vi "CPP_SpectraFit.vi"() -> (5 "Plug in titles":string[](array[string]), 7 "Plug in values":string[](array[string]))   [LabVIEW 2010]
uses:
  Controls/Instrument_Array.ctl
  Controls/Post_Process.ctl
  Controls/Graph_Type.ctl
  Globals/Meas_global.vi
  Globals/Plug_in_data_global.vi
panel:
  out "dF/ Hz":dbl
  in  "Show Smooth":bool=TRUE
  in  "Save Spectra?":bool
  in  "Desired number of samples per block":i32=32767
  in  "Calculate Spectra and Histogram?":bool=TRUE
  out "Spectra":cluster{dbl, dbl, "Spectrum output array":dbl[]}(graph)
  in  "Averaging samples":i32=1 min=1 max=1000
  in  "Spectra Index (from ALL channels)":i32
  out "Waveform Graph":dbl[][](graph)
  in  "Channels to Plot":i32[](array[ring])=[0] items=["Pitot (Uref)", "HW (Uhw)", "Gen (Trav)", "Save Nothing"]
  # "Run this VI to update the channel names"
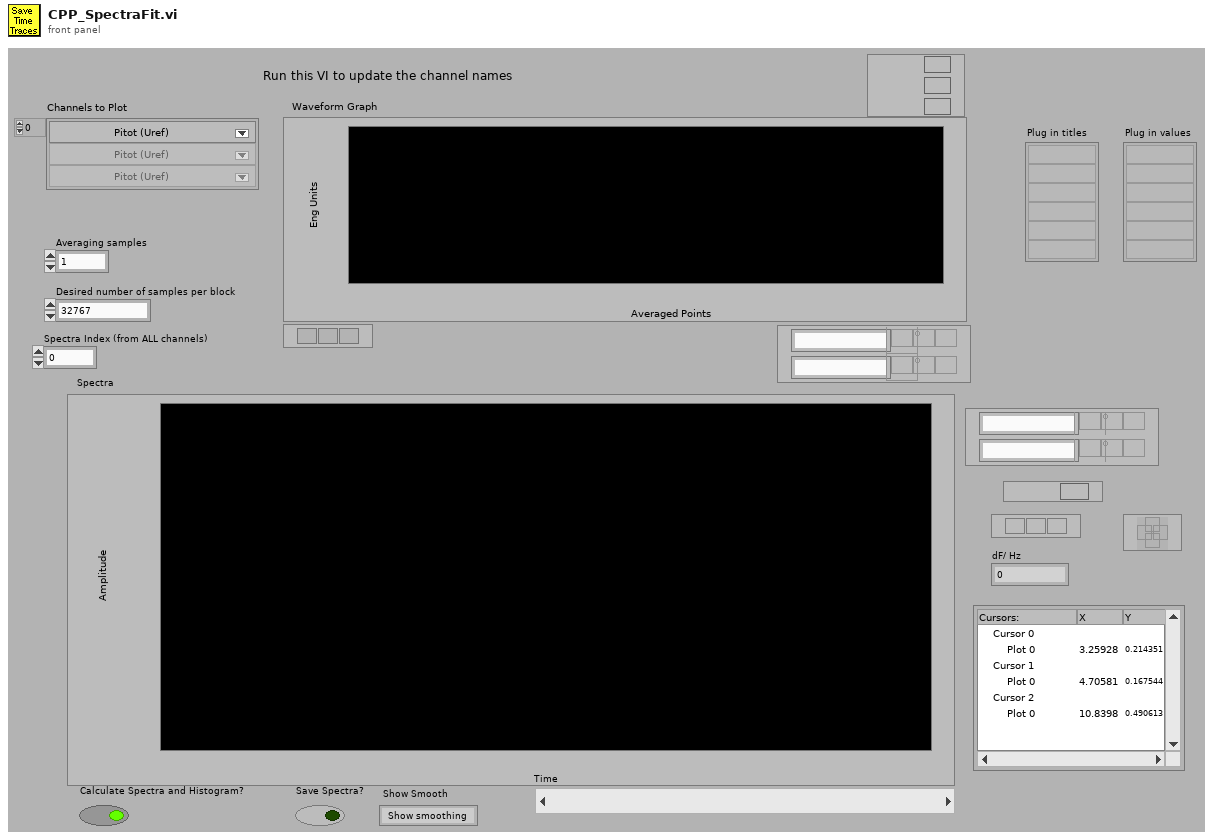
[diagram p1: front panel]
types:
  T1 = typedef "Analysis_info_cluster.ctl" = cluster{"Colour":u32, "Inst type":T2, "Inst name":string, "Symbol":string, "Code name":string, "Extra Info":string, "Inst Array":T3, "Index":i32, "Voltage Index":i32, "Extra Titles":string[], "Extra Values":string[]}
  T2 = typedef "Inst_type.ctl" = enum16{"Propeller anemometer", "Raw voltage", "Pressure Transducer", "Pitot-static tube", "Preston tube", "Hot wire", "Cross wire 1", "Cross wire 2", "Generic Linear", "Generic Polynomial", "Generic BackPoly", "Fast FID", "Thermocouple", "Cold wire", "Pulsed Wire", "LDA Vel", "LDA Tran time", "LDA Arr time"}
  T3 = typedef "Instrument_Array.ctl" = enum16{"PWA", "LDA", "Analogue"}
  T4 = typedef "Post_Process.ctl" = enum16{"Take New Data", "Post Process Raw Data File"}
  T5 = typedef "Graph_Type.ctl" = enum16{"Show no graph", "Voltage trace", "Velocity trace", "Vel histogram", "Spectrum", "f.E(f) v Log f", "Auto-Corr"}
  T6 = cluster{"Plot 1":u16, "Plot 2":u16, "Save graph":u16, "Plot Type":T5}
  T7 = cluster{dbl, dbl, "Spectrum output array":dbl[]}[]
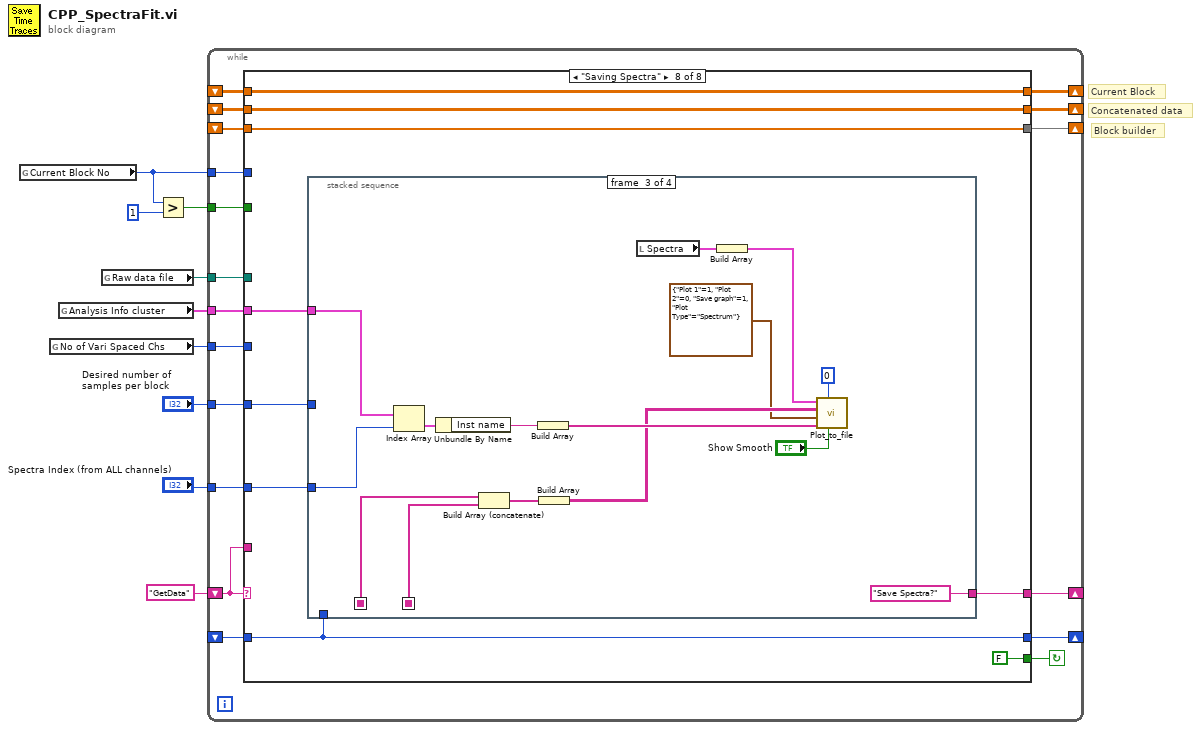
[diagram p0: block diagram]
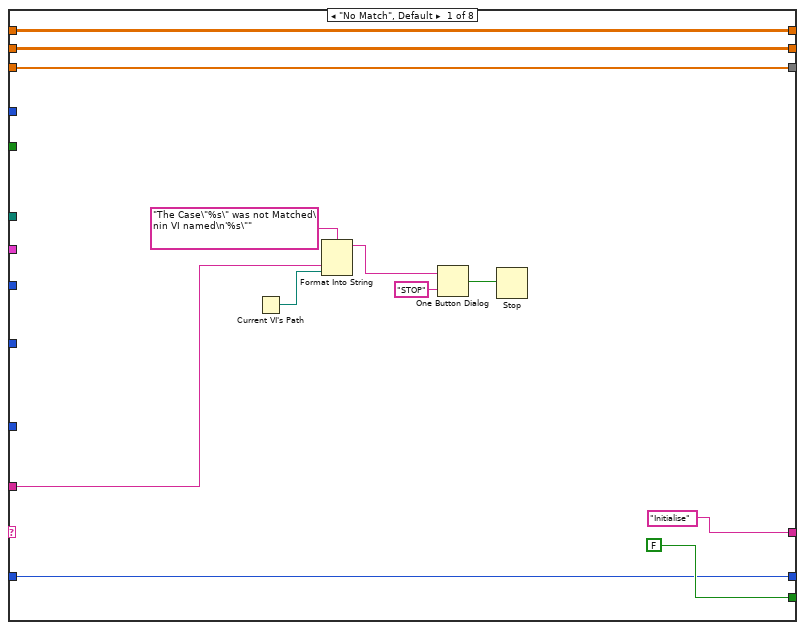
[diagram p2: hidden frame]
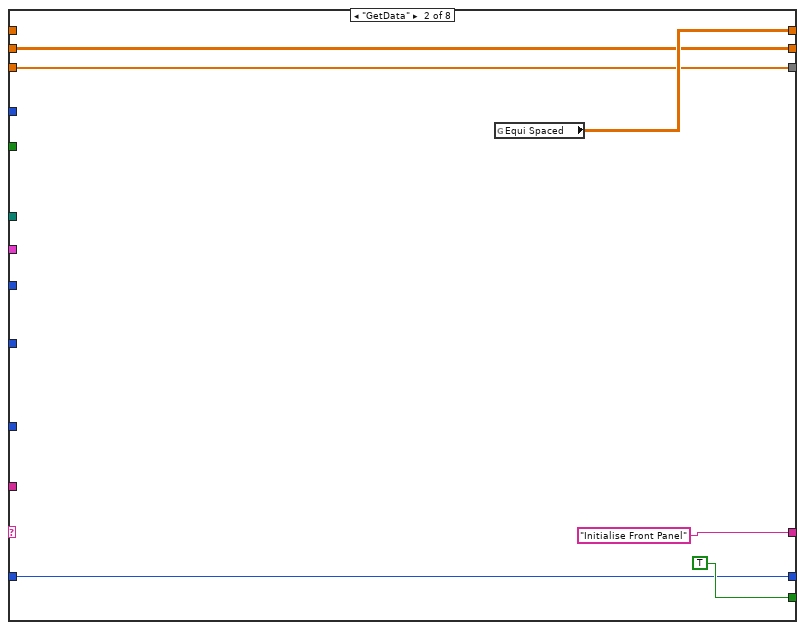
[diagram p3: hidden frame]
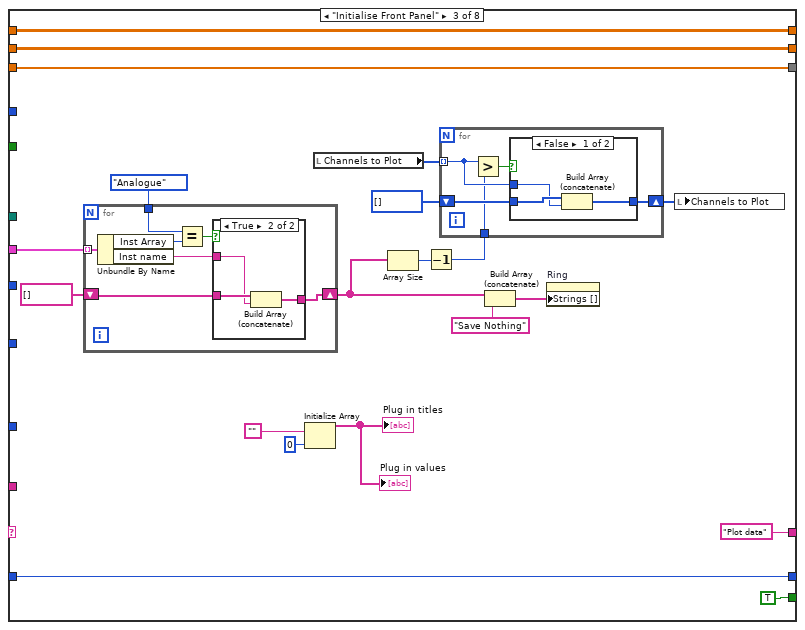
[diagram p4: hidden frame]
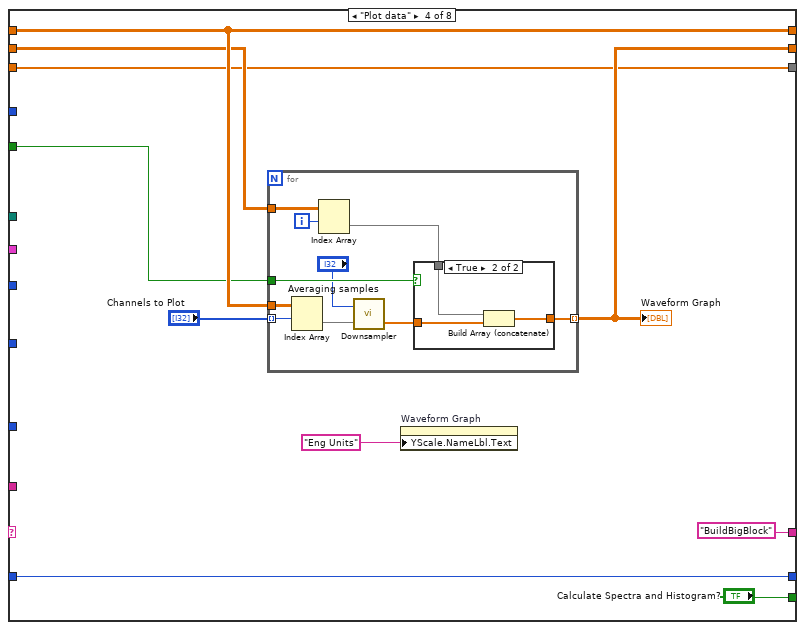
[diagram p7: hidden frame]
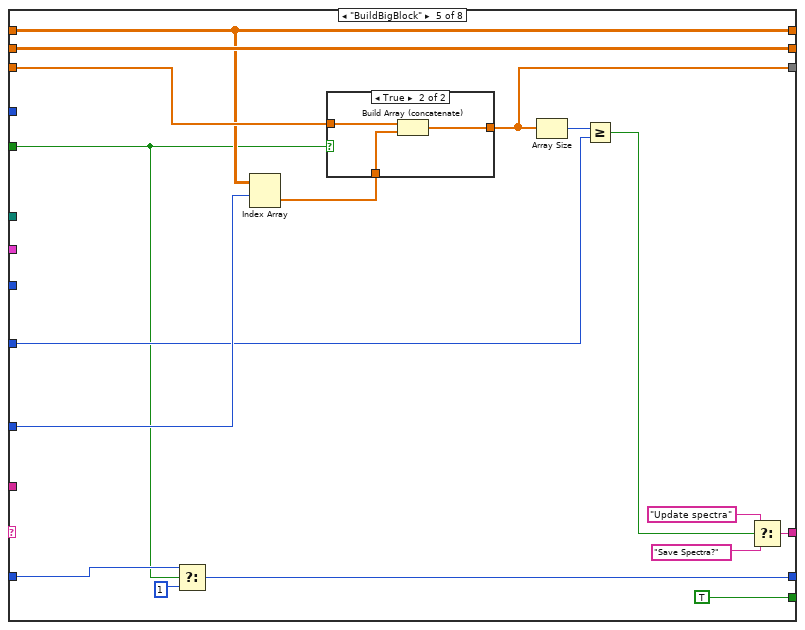
[diagram p9: hidden frame]
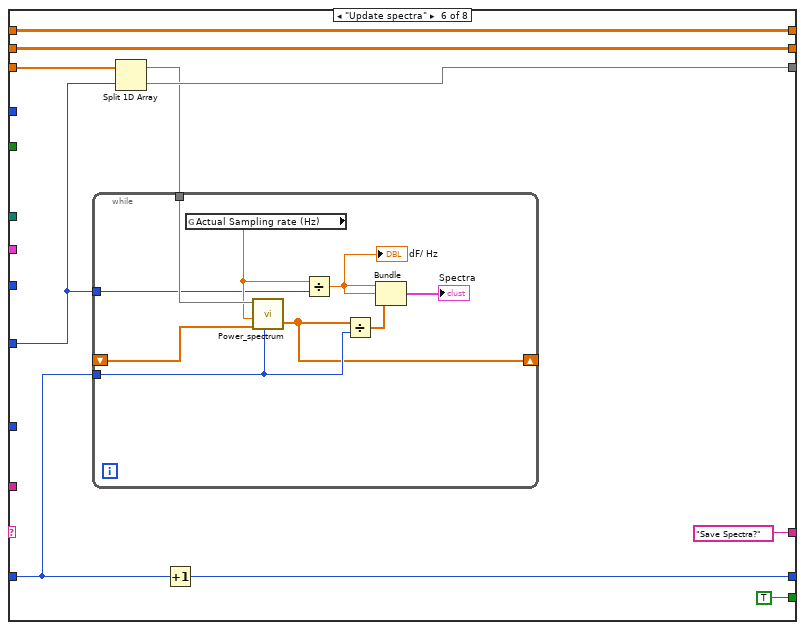
[diagram p11: hidden frame]
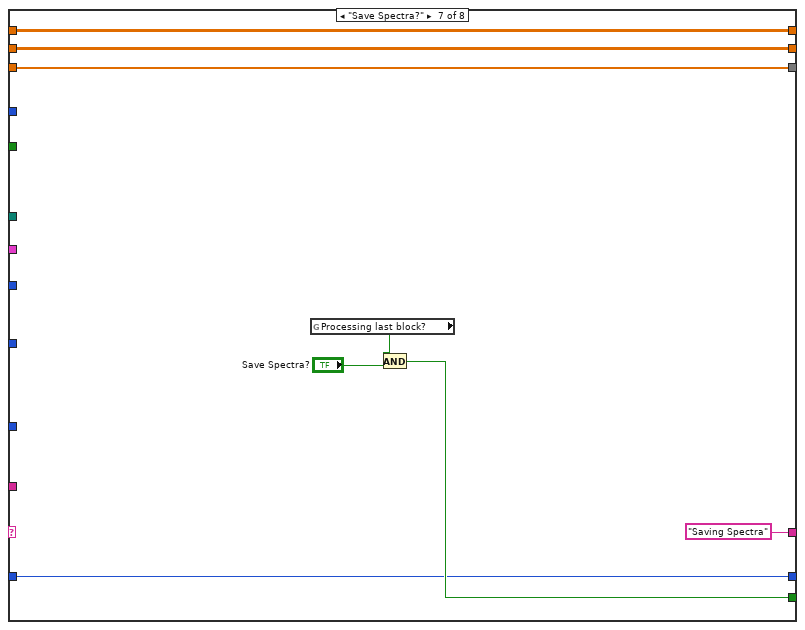
[diagram p12: hidden frame]
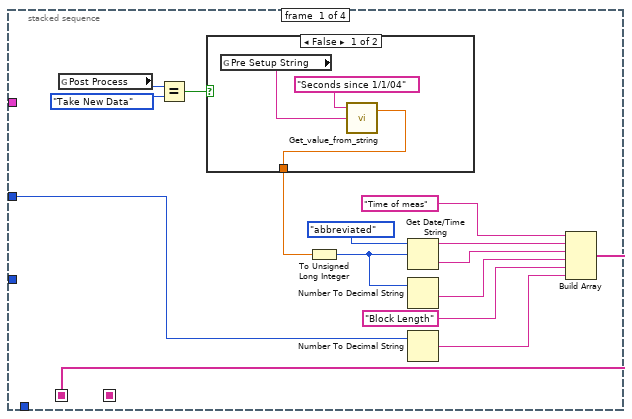
[diagram p13: hidden frame]
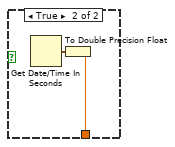
[diagram p14: hidden frame]
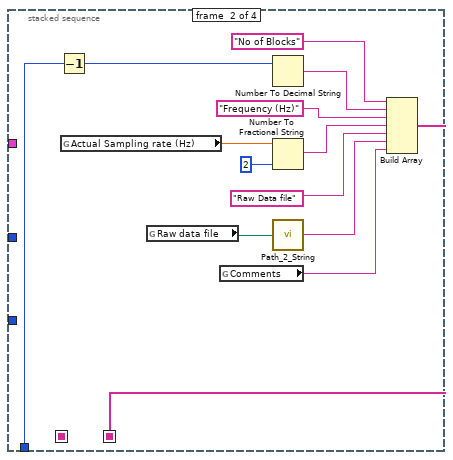
[diagram p15: hidden frame]
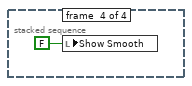
[diagram p16: hidden frame]
diagram:
  # "Block builder"
  # "Concatenated data"
  # "Current Block"
  n1 = global read "Meas_global.vi" "Current Block No"() -> (w6:i32)
  n2 = global read "Meas_global.vi" "No of Vari Spaced Chs"() -> (w4:i32)
  n3 = global read "Meas_global.vi" "Analysis Info cluster"() -> (w5:T1[])
  n4 = global read "Meas_global.vi" "Raw data file"() -> (w8:path)
  n5 = Greater?(x=w6, y=1) -> (0:w3:bool)
  n6 = while {
    shift-left: "GetData" -> [w25]
    shift-right: [w26] -> _
    tunnel: w8 -> [w24]
    tunnel: w3 -> [w23]
    tunnel: w6 -> [w22]
    tunnel: w5 -> [w21]
    tunnel: w4 -> [w20]
    shift-right: [w19] -> _
    shift-left: _ -> [w18]
    shift-right: [w16] -> _
    shift-left: _ -> [w17]
    shift-right: [w14] -> _
    shift-left: _ -> [w15]
    tunnel: "Desired number of samples per block" -> [w13]
    tunnel: "Spectra Index (from ALL channels)" -> [w12]
    shift-right: [w11] -> _
    shift-left: _ -> [w10]
    stop <- w27 continue-if-true
    n7 = case shown="\"Saving Spectra\"" w25 {
      tunnel: [FALSE TRUE TRUE "Calculate Spectra and Histogram?" TRUE ("Calculate Spectra and Histogram?") TRUE ("Calculate Spectra and Histogram?") w152 FALSE ("Calculate Spectra and Histogram?")] -> w27
      tunnel: ["Initialise" "Initialise Front Panel" "Plot data" "BuildBigBlock" ("t") w111 "Save Spectra?" "Saving Spectra" w165] -> w26
      tunnel: w25 -> [w34 _ _ _ _ _ _ _]
      tunnel: w24 -> [_ _ _ _ _ _ _ _]
      tunnel: w23 -> [_ _ _ w93 w114 _ _ _]
      tunnel: w22 -> [_ _ _ _ _ _ _ _]
      tunnel: w21 -> [_ _ w49 _ _ _ _ w163]
      tunnel: w20 -> [_ _ _ _ _ _ _ _]
      tunnel: [w31 w43 w55 w95 w124 w139 w157 w166] -> w19
      tunnel: w18 -> [w31 _ w55 w95 w124 w139 w157 w166]
      tunnel: w17 -> [w30 w42 w54 w94 w125 w140 w158 w167]
      tunnel: [w30 w42 w54 w91 w125 w140 w158 w167] -> w16
      tunnel: w15 -> [w29 w41 w51 w88 w126 w138 w155 w164]
      tunnel: [w29 w41 w51 w88 w122 w137 w155 w164] -> w14
      tunnel: w13 -> [_ _ _ _ w118 w133 _ w160]
      tunnel: w12 -> [_ _ _ _ w120 _ _ w162]
      tunnel: [w28 w40 w50 w87 w115 w131 w151 w159] -> w11
      tunnel: w10 -> [w28 w40 w50 w87 w116 w132 w151 w159]
      frame "No Match", Default {
        n8 = Current VI's Path() -> (path=w33:path)
        n9 = Format Into String(format string="The Case\"%s\" was not Matched\nin VI named\n'%s\"" ("Format String"), w34, w33) -> (resulting string=w37:string)  [unwired: 2 in, 1 out]
        n10 = One Button Dialog(message=w37, button name ("OK")="STOP") -> (true=w35:bool)
        n11 = Stop(stop? (T)=w35) -> ()
      }
      frame "GetData" {
        n12 = global read "Plug_in_data_global.vi" "Equi Spaced"() -> (w43:dbl[][])
      }
      frame "Initialise Front Panel" {
        n13 = for {
          tunnel: Instrument_Array."Analogue" ("Inst Array") -> [w71]
          tunnel: w49 -> [w70] mode=indexing
          shift-right: [w67] -> w48
          shift-left: string[] [] -> [w68]
          n14 = Unbundle By Name(w70) -> ("Inst Array"=w72:T3, "Inst name"=w66:string)
          n15 = Equal?(x=w71, y=w72) -> (x = y?=w69:bool)
          n16 = case shown="True" w69 {
            tunnel: w68 -> [w73 w76]
            tunnel: [w73 w75] -> w67
            tunnel: w66 -> [_ w74]
            frame False {
            }
            frame True {
              n17 = Build Array (concatenate)(w76, w74) -> (w75:string[])
            }
          }
        }
        n18 = Initialize Array("", 0) -> (→"Plug in values" →"Plug in titles":string[])
        n19 = local read "Channels to Plot"() -> (w62:i32[])
        n20 = Array Size(array=w48) -> (size(s)=w57:i32)
        n21 = Decrement(x=w57) -> (x-1=w56:i32)
        n22 = for {
          tunnel: w62 -> [w78] mode=indexing
          shift-right: [w79] -> w60
          shift-left: i32[] [] -> [w80]
          tunnel: w56 -> [w77]
          n23 = Greater?(x=w78, y=w77) -> (0:w81:bool)
          n24 = case shown="False" w81 {
            tunnel: w80 -> [w84 w85]
            tunnel: [w83 w85] -> w79
            tunnel: w78 -> [w82 _]
            frame False {
              n25 = Build Array (concatenate)(w84, w82) -> (w83:i32[])
            }
            frame True {
            }
          }
        }
        n26 = Build Array (concatenate)(w48, "Save Nothing") -> (w58:string[])
        n27 = property on="Ring" class="Ring (strict)"("Strings []"=w58) -> ()  [unwired: 2 in, 2 out]
        n28 = local write "Channels to Plot"(w60) -> ()
      }
      frame "Plot data" {
        n29 = for {
          tunnel: w95 -> [w105]
          tunnel: "Channels to Plot" -> [w104] mode=indexing
          tunnel: w94 -> [w101]
          tunnel: [w102] -> w91 mode=indexing
          tunnel: w93 -> [w103]
          i -> [w100]
          n30 = Index Array(array=w105, index (row)=w104) -> (element=w98:dbl[])  [unwired: 1 in]
          n31 = Index Array(array=w101, index (row)=w100) -> (element=w99:dbl[])  [unwired: 1 in]
          n32 = call "Downsampler.vi"("Input Array"=w98, "Averaging samples"="Averaging samples") -> ("Downsampled Array"=w97:dbl[])  [unwired: 1 out]
          n33 = case shown="True" w103 {
            tunnel: w99 -> [_ w109]
            tunnel: w97 -> [w106 w108]
            tunnel: [w106 w107] -> w102
            frame False {
            }
            frame True {
              n34 = Build Array (concatenate)(w109, w108) -> (w107:dbl[])
            }
          }
        }
        "Waveform Graph" <- w91
        n35 = property on="Waveform Graph" class="WFGraph (strict)"("YScale.NameLbl.Text"="Eng Units") -> ()  [unwired: 2 in, 2 out]
      }
      frame "BuildBigBlock" {
        n36 = Select(t=w116, s=w114, f=1) -> (s? t:f=w115:i32)
        n37 = Index Array(array=w124, index (row)=w120) -> (element=w123:dbl[])  [unwired: 1 in]
        n38 = case shown="True" w114 {
          tunnel: w126 -> [_ w130]
          tunnel: [w127 w129] -> w122
          tunnel: w123 -> [w127 w128]
          frame False {
          }
          frame True {
            n39 = Build Array (concatenate)(w130, w128) -> (w129:dbl[])
          }
        }
        n40 = Array Size(array=w122) -> (size(s)=w121:i32)
        n41 = Greater Or Equal?(x=w121, y=w118) -> (x >= y?=w110:bool)
        n42 = Select(t="Update spectra", s=w110, f="Save Spectra?") -> (s? t:f=w111:string)
      }
      frame "Update spectra" {
        n43 = Split 1D Array(array=w138, index=w133) -> (first subarray=w134:dbl[], second subarray=w137:dbl[])
        n44 = while {
          shift-left: _ -> [w148]
          shift-right: [w141] -> _
          tunnel: w134 -> [w149]
          tunnel: w132 -> [w147]
          tunnel: w133 -> [w145]
          stop <- FALSE continue-if-true
          n45 = global read "Meas_global.vi" "Actual Sampling rate (Hz)"() -> (w146:dbl)
          n46 = call "Power_spectrum.vi"("U"=w149, "Sampling frequency"=w146, "Spectrum input array"=w148, "Block No"=w147) -> ("Spectrum output array"=w141:dbl[])  [unwired: 1 in, 1 out]
          n47 = Divide(x=w146, y=w145) -> (x/y=w143:dbl)
          "dF/ Hz" <- w143
          n48 = Divide(x=w141, y=w147) -> (x/y=w142:dbl[])
          n49 = Bundle(w143, w143, w142) -> (→"Spectra":cluster{dbl, dbl, dbl[]})  [unwired: 1 out]
        }
        n50 = Increment(x=w132) -> (x+1=w131:i32)
      }
      frame "Save Spectra?" {
        n51 = global read "Meas_global.vi" "Processing last block?"() -> (w153:bool)
        n52 = And(x=w153, y="Save Spectra?") -> (x .and. y?=w152:bool)
      }
      frame "Saving Spectra" {
        n53 = stacked-sequence {
          seq-local: [w171 _ _ _] -> [_ _ w204 _]
          seq-local: [_ w191 _ _] -> [_ _ w203 _]
          tunnel: [_ _ "Save Spectra?" _] -> w165
          tunnel: w163 -> [_ _ w210 _]
          tunnel: w162 -> [_ _ w209 _]
          tunnel: w160 -> [w169 _ _ _]
          tunnel: w159 -> [_ w189 _ _]
          frame #0 {
            n54 = global read "Meas_global.vi" "Post Process"() -> (w173:T4)
            n55 = Equal?(x=w173, y=Post_Process."Take New Data" ("Post Process")) -> (x = y?=w174:bool)
            n56 = case shown="False" w174 {
              tunnel: [w182 w186] -> w175
              frame False {
                n57 = global read "Meas_global.vi" "Pre Setup String"() -> (w183:string)
                n58 = call "Get_value_from_string.vi"("Input string"=w183, "Variable name"="Seconds since 1/1/04") -> ("Value"=w182:dbl)  [unwired: 1 in, 1 out]
              }
              frame True {
                n59 = Get Date/Time In Seconds() -> (seconds since 1Jan1904=w185:timestamp)
                n60 = To Double Precision Float(number=w185) -> (double precision float=w186:dbl)
              }
            }
            n61 = To Unsigned Long Integer(number=w175) -> (unsigned 32bit integer=w179:u32)
            n62 = Get Date/Time String(date format (0)=enum16{"short", "long", "abbreviated"}."abbreviated", seconds (now)=w179) -> (date string=w177:string, time string=w178:string)  [unwired: 1 out]
            n63 = Number To Decimal String(number=w179) -> (decimal integer string=w180:string)  [unwired: 1 out]
            n64 = Number To Decimal String(number=w169) -> (decimal integer string=w168:string)  [unwired: 1 out]
            n65 = Build Array("Time of meas", w177, w178, w180, "Block Length" ("element"), w168) -> (w171:string[])
          }
          frame #1 {
            n66 = Decrement(x=w189) -> (x-1=w188:i32)
            n67 = global read "Meas_global.vi" "Actual Sampling rate (Hz)"() -> (w192:dbl)
            n68 = global read "Meas_global.vi" "Raw data file"() -> (w198:path)
            n69 = global read "Meas_global.vi" "Comments"() -> (w197:string)
            n70 = Number To Decimal String(number=w188) -> (decimal integer string=w187:string)  [unwired: 1 out]
            n71 = Number To Fractional String(number=w192, precision (6)=i16 2) -> (F-format string=w195:string)  [unwired: 2 out]
            n72 = call "Path_2_String.vi"("Real Path"=w198) -> ("Path String"=w199:string)
            n73 = Build Array("No of Blocks", w187, "Frequency (Hz)", w195, "Raw Data file", w199, w197) -> (w191:string[])
          }
          frame #2 {
            n74 = Index Array(array=w210, index=w209) -> (element=w208:T1)
            n75 = Unbundle By Name(w208) -> ("Inst name"=w207:string)
            n76 = Build Array (concatenate)(w204, w203) -> (w202:string[])
            n77 = Build Array(w207) -> (w206:string[])
            n78 = Build Array(w202) -> (w201:string[][])
            n79 = local read "Spectra"() -> (w213:cluster{dbl, dbl, "Spectrum output array":dbl[]})
            n80 = Build Array(w213) -> (w212:T7)
            n81 = call "Plot_to_file.vi"("Show Smooth"="Show Smooth", "Start trace No"=0, "Trace names"=w206, "Graph"=T6 {"Plot 1"=1, "Plot 2"=0, "Save graph"=1, "Plot Type"=enum."Spectrum"}, "Plot file label"=w201, "Plot data"=w212) -> ()  [unwired: 6 out]
          }
          frame #3 {
            n82 = local write "Show Smooth"(FALSE ("Show Smooth")) -> ()
          }
        }
      }
    }
  }
